vi "rad_Get Backplane Type.vi"(8 "error in (no error)":errorcluster, 11 "Controller IP":string) -> (0 "error out":errorcluster, 2 "Backplane Type":string, 3 "Controller IP Out":string)   [LabVIEW 2020]
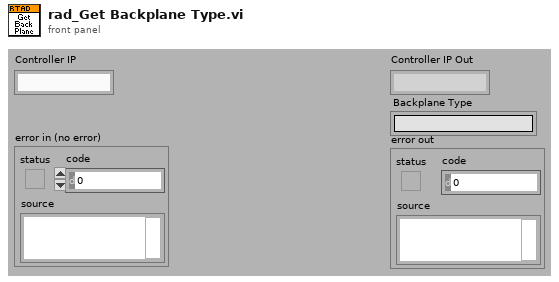
[diagram p1: front panel]
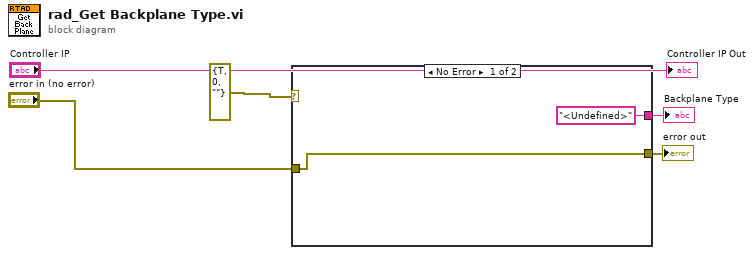
[diagram p0: block diagram]
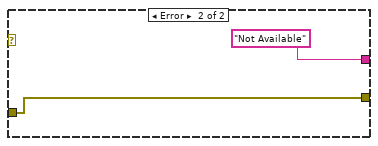
[diagram p2: hidden frame]
diagram:
  n1 = case shown="No Error" errorcluster {"status"=TRUE, "code"=0, "source"=""} ("error out") {
    tunnel: ["<Undefined>" "Not Available"] -> w2
    tunnel: [w7 w9] -> w1
    tunnel: "error in (no error)" -> [w7 w9]
    frame No Error {
    }
    frame Error {
    }
  }
  "Backplane Type" <- w2
  "error out" <- w1
  "Controller IP Out" <- "Controller IP"
